vi "Display Data.vi"(8 "Error In":errorcluster, 11 "Numeric in":refnum<class "Numeric.lvclass">) -> (0 "Error Out":errorcluster, 3 "Numeric out":refnum<class "Numeric.lvclass">)   [LabVIEW 2023, in "Numeric.lvclass"]
doc: "The method displays the received data of numeric data type."
uses:
  Numeric.lvclass
  Numeric.lvclass/Numeric.ctl
panel:
  out "Numeric Data":dbl
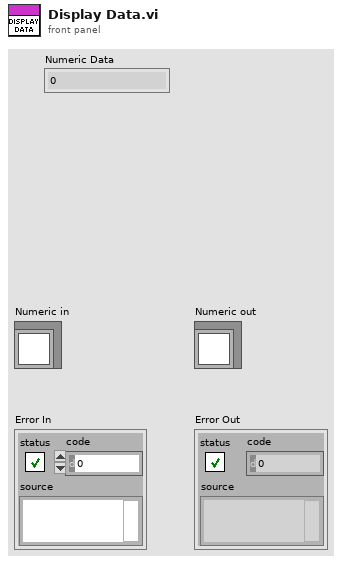
[diagram p1: front panel]
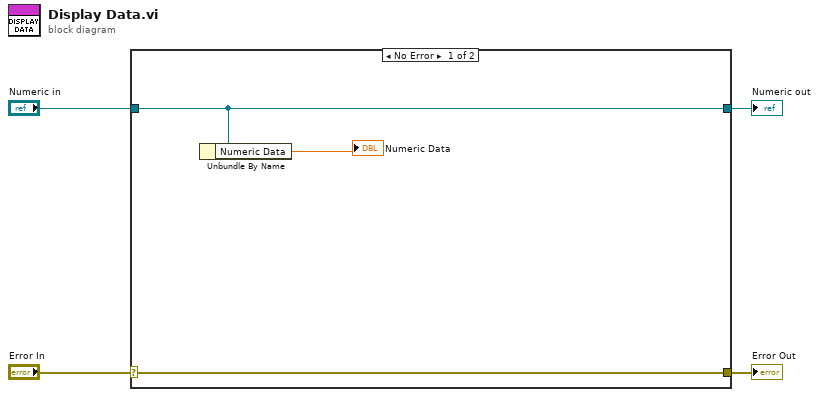
[diagram p0: block diagram]
diagram:
  n1 = case shown="No Error" "Error In" {
    selector: "Error In" -> [w7 w9]
    tunnel: [w7 w9] -> w3
    tunnel: [w6 w8] -> w1
    tunnel: "Numeric in" -> [w6 w8]
    frame No Error {
      n2 = Unbundle By Name(w6) -> ("Numeric Data"=→"Numeric Data":dbl)
    }
    frame Error {
    }
  }
  "Error Out" <- w3
  "Numeric out" <- w1
